vi "terminate.vi"(8 "error in (no error)":errorcluster, 11 "DL090623TwoDAnalyser in":refnum<class "AnalyserDL090623TwoD.lvclass">) -> (0 "error out":errorcluster, 3 "DL090623TwoDAnalyser out":refnum<class "AnalyserDL090623TwoD.lvclass">)   [LabVIEW 2010, in "AnalyserDL090623TwoD.lvclass"]
doc: "The dynamic dispatch version of this VI terminates the plug-in object by releasing all of its resources."
uses:
  AnalyserDL090623TwoD.lvclass
  common/classes/Image/Image/Image.lvclass
  Segmenter/GenericSegmenter/GenericSegmenter/GenericSegmenter.lvclass
  TraceProcessor/GenericTraceProcessor/GenericTraceProcessor/GenericTraceProcessor.lvclass
  AnalyserDL090624Scaffold/AnalyserDL090624Scaffold/AnalyserDL090624Scaffold.lvclass
  common/classes/ErrorController/ErrorController/ErrorController.lvclass
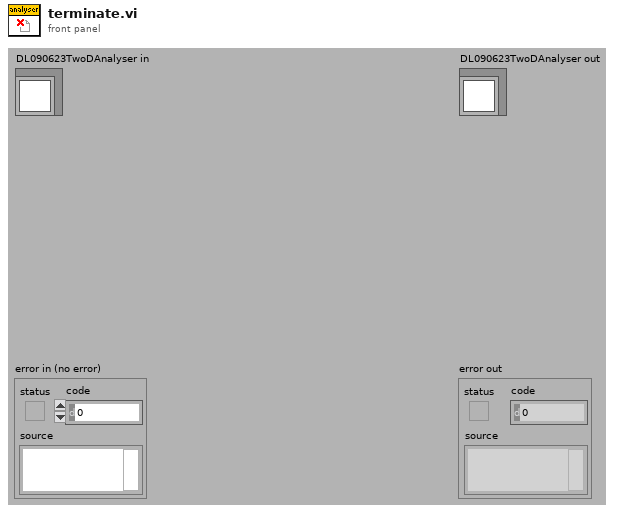
[diagram p1: front panel]
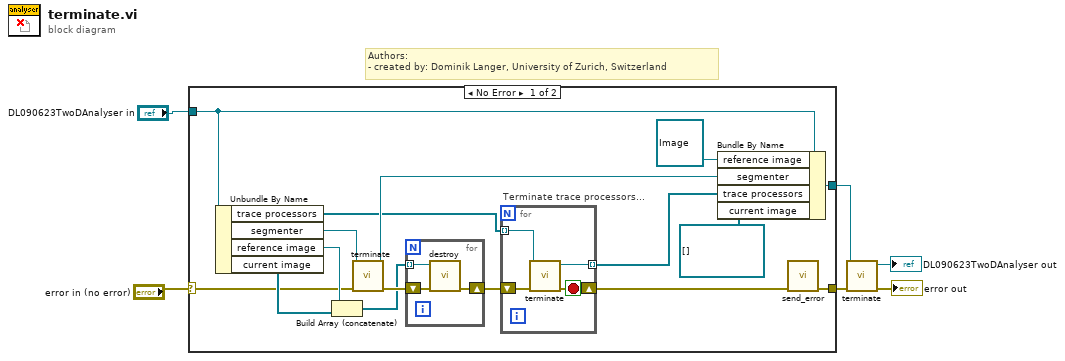
[diagram p0: block diagram]
diagram:
  # "Authors: \n- created by: Dominik Langer, University of Zurich, Switzerland"
  n1 = case shown="No Error" "error in (no error)" {
    selector: "error in (no error)" -> [w8 w30]
    tunnel: "DL090623TwoDAnalyser in" -> [w16 w31]
    tunnel: [w17 w30] -> w2
    tunnel: [w22 w31] -> w1
    frame No Error {
      n2 = Unbundle By Name(w16) -> ("trace processors"=w7:refnum<class "GenericTraceProcessor.lvclass">[], "segmenter"=w21:refnum<class "GenericSegmenter.lvclass">, "reference image"=w15:refnum<class "Image.lvclass">, "current image"=w14:refnum<class "Image.lvclass">[])
      n3 = Build Array (concatenate)(w15, w14) -> (w9:refnum<class "Image.lvclass">[])
      n4 = call-dynamic "terminate.vi"("error in (no error)"=w8, "GenericPlugin in"=w21) -> ("error out"=w11:errorcluster, "GenericPlugin out"=w20:refnum<class "GenericSegmenter.lvclass">)  [unwired: 8 out]
      n5 = for {
        shift-right: [w24] -> w10
        shift-left: w11 -> [w25]
        tunnel: w9 -> [w23] mode=indexing
        n6 = call-dynamic "destroy.vi"("error in (no error)"=w25, "Image in"=w23) -> ("error out"=w24:errorcluster)  [unwired: 9 out]
      }
      n7 = for "Terminate trace processors..." {
        tunnel: w7 -> [w29] mode=indexing
        tunnel: [w27] -> w19 mode=indexing
        shift-right: [w26] -> w18
        shift-left: w10 -> [w28]
        stop <- w26 stop-if-true
        n8 = call-dynamic "terminate.vi"("error in (no error)"=w28, "GenericPlugin in"=w29) -> ("error out"=w26:errorcluster, "GenericPlugin out"=w27:refnum<class "GenericTraceProcessor.lvclass">)  [unwired: 8 out]
      }
      n9 = Bundle By Name(cluster=w16, "reference image"=refnum<class "Image.lvclass"> refnum ("Image.lvclass"), "segmenter"=w20, "trace processors"=w19, "current image"=refnum<class "Image.lvclass">[] []) -> (w22:refnum<class "AnalyserDL090623TwoD.lvclass">)
      n10 = call "send_error.vi"("error in (no error)"=w18) -> ("error out"=w17:errorcluster)  [unwired: 10 in]
    }
    frame Error {
    }
  }
  n11 = call-parent "terminate.vi"("error in (no error)"=w2, "GenericPlugin in"=w1) -> ("error out"=→"error out":errorcluster, "GenericPlugin out"=→"DL090623TwoDAnalyser out":refnum<class "AnalyserDL090623TwoD.lvclass">)  [unwired: 8 out]
